vi "Import Structure from DB.vi"(8 "error in (no error)":errorcluster, 10 "Structure ID":string, 11 "connection reference":T2) -> (0 "error out":errorcluster, 2 "Loaded Structure":T1={"Structure Name"="Batch6_3+111 Quasi-Bulk", "Lattice vector a"=[9.1641, 0.0, 0.0], "Lattice vector b"=[0.0, 7.93635, 0.0], "Lattice vector c"=[0.0, 0.0, 53.7091], "Atoms Array"=[{"Atom Name"="", "Positions (Direct)"=[[0.036896, 0.129554, 0.035254], [0.536896, 0.129554, 0.035254], [0.286896, 0.629554, 0.035254], [0.786896, 0.629554, 0.035254], [0.285415, 0.295133, 0.107673], [0.785415, 0.295133, 0.107673], [0.035415, 0.795133, 0.107673], [0.535415, 0.795133, 0.107673], [0.033615, 0.463308, 0.180101], [0.533615, 0.463308, 0.180101], [0.283615, 0.963308, 0.180101], [0.783615, 0.963308, 0.180101], [0.030844, 0.131453, 0.252535], [0.530844, 0.131453, 0.252535], [0.280844, 0.631453, 0.252535], [0.780844, 0.631453, 0.252535], [0.278379, 0.302058, 0.324923], [0.778379, 0.302058, 0.324923], [0.028379, 0.802058, 0.324923], [0.528379, 0.802058, 0.324923], [0.031198, 0.471844, 0.397363], [0.531198, 0.471844, 0.397363], [0.281198, 0.971844, 0.397363], [0.781198, 0.971844, 0.397363], [0.03247, 0.140643, 0.469814], [0.53247, 0.140643, 0.469814], [0.28247, 0.640643, 0.469814], [0.78247, 0.640643, 0.469814], [0.284308, 0.303948, 0.542263], [0.784308, 0.303948, 0.542263], [0.034308, 0.803948, 0.542263], [0.534308, 0.803948, 0.542263], [0.035944, 0.468219, 0.614701], [0.535944, 0.468219, 0.614701], [0.285944, 0.968219, 0.614701], [0.785944, 0.968219, 0.614701], [0.037813, 0.131858, 0.687216], [0.537813, 0.131858, 0.687216], [0.787813, 0.631858, 0.687216], [0.287813, 0.631858, 0.687216], [0.038238, 0.463759, 0.759817], [0.538238, 0.463759, 0.759817], [0.288238, 0.963758, 0.759817], [0.788238, 0.963758, 0.759817], [0.038639, 0.130134, 0.831025], [0.538639, 0.130134, 0.831025], [0.288639, 0.630134, 0.831025], [0.788639, 0.630134, 0.831025], [0.285712, 0.295024, 0.89873], [0.785712, 0.295024, 0.89873], [0.035712, 0.795024, 0.89873], [0.535712, 0.795024, 0.89873], [0.032596, 0.464879, 0.966384], [0.532596, 0.464879, 0.966384], [0.282596, 0.964879, 0.966384], [0.782596, 0.964879, 0.966384]], "Positions (Cartesian)"=[[0.33811863359999994, 1.0281858879, 1.8934606114], [4.9201686336, 1.0281858879, 1.8934606114], [2.6291436335999996, 4.9963608879, 1.8934606114], [7.2111936336, 4.9963608879, 1.8934606114], [2.6155716014999997, 2.34227878455, 5.7830199243000004], [7.197621601499999, 2.34227878455, 5.7830199243000004], [0.3245466015, 6.31045378455, 5.7830199243000004], [4.9065966014999995, 6.31045378455, 5.7830199243000004], [0.30805122149999997, 3.6769744458, 9.673062619100001], [4.890101221499999, 3.6769744458, 9.673062619100001], [2.5990762215, 7.6451494458, 9.673062619100001], [7.1811262215, 7.6451494458, 9.673062619100001], [0.2826575004, 1.04325701655, 13.5634275685], [4.8647075004, 1.04325701655, 13.5634275685], [2.5736825004, 5.011432016550001, 13.5634275685], [7.155732500399999, 5.011432016550001, 13.5634275685], [2.5510929938999998, 2.3972380083, 17.4513218993], [7.1331429939, 2.3972380083, 17.4513218993], [0.2600679939, 6.3654130083, 17.4513218993], [4.8421179939000005, 6.3654130083, 17.4513218993], [0.28590159179999997, 3.7447191294, 21.3420091033], [4.867951591799999, 3.7447191294, 21.3420091033], [2.5769265918, 7.7128941294, 21.3420091033], [7.158976591799999, 7.7128941294, 21.3420091033], [0.29755832699999996, 1.11619207305, 25.2332871074], [4.879608327, 1.11619207305, 25.2332871074], [2.588583327, 5.08436707305, 25.2332871074], [7.170633327, 5.08436707305, 25.2332871074], [2.6054269428, 2.4122377098, 29.124457693300002], [7.1874769428, 2.4122377098, 29.124457693300002], [0.31440194279999994, 6.3804127098, 29.124457693300002], [4.8964519428, 6.3804127098, 29.124457693300002], [0.32939441039999995, 3.71594986065, 33.0150374791], [4.9114444104, 3.71594986065, 33.0150374791], [2.6204194104, 7.684124860650001, 33.0150374791], [7.202469410399999, 7.684124860650001, 33.0150374791], [0.3465221133, 1.0464712383, 36.909752865600005], [4.9285721133, 1.0464712383, 36.909752865600005], [7.2195971133, 5.0146462383, 36.909752865600005], [2.6375471132999997, 5.0146462383, 36.909752865600005], [0.3504168558, 3.6805537396499997, 40.809087234699994], [4.9324668557999995, 3.6805537396499997, 40.809087234699994], [2.6414418557999997, 7.6487208033, 40.809087234699994], [7.2234918558, 7.6487208033, 40.809087234699994], [0.35409165989999997, 1.0327889709, 44.6336048275], [4.9361416599, 1.0327889709, 44.6336048275], [2.6451166599, 5.0009639709, 44.6336048275], [7.227166659899999, 5.0009639709, 44.6336048275], [2.6182933392, 2.3414137224, 48.269979443000004], [7.200343339199999, 2.3414137224, 48.269979443000004], [0.3272683392, 6.3095887224, 48.269979443000004], [4.9093183391999995, 6.3095887224, 48.269979443000004], [0.29871300359999997, 3.6894424516499997, 51.9036148944], [4.880763003599999, 3.6894424516499997, 51.9036148944], [2.5897380036, 7.65761745165, 51.9036148944], [7.171788003599999, 7.65761745165, 51.9036148944]]}, {"Atom Name"="", "Positions (Direct)"=[[0.286795, 0.296109, 0.054458], [0.786795, 0.296109, 0.054458], [0.036795, 0.796109, 0.054458], [0.536795, 0.796109, 0.054458], [0.035258, 0.462031, 0.126878], [0.535258, 0.462031, 0.126878], [0.285258, 0.962031, 0.126878], [0.785258, 0.962031, 0.126878], [0.033445, 0.130094, 0.199309], [0.533445, 0.130094, 0.199309], [0.283445, 0.630094, 0.199309], [0.783445, 0.630094, 0.199309], [0.280766, 0.298203, 0.27171], [0.780766, 0.298203, 0.27171], [0.030766, 0.798203, 0.27171], [0.530766, 0.798203, 0.27171], [0.028505, 0.468822, 0.344121], [0.528505, 0.468822, 0.344121], [0.278505, 0.968822, 0.344121], [0.778505, 0.968822, 0.344121], [0.03126, 0.138635, 0.416572], [0.53126, 0.138635, 0.416572], [0.28126, 0.638635, 0.416572], [0.78126, 0.638635, 0.416572], [0.282556, 0.307128, 0.489026], [0.782556, 0.307128, 0.489026], [0.032556, 0.807128, 0.489026], [0.532556, 0.807128, 0.489026], [0.034374, 0.470438, 0.56147], [0.534374, 0.470438, 0.56147], [0.284374, 0.970438, 0.56147], [0.784374, 0.970438, 0.56147], [0.035964, 0.134698, 0.633895], [0.535964, 0.134698, 0.633895], [0.285964, 0.634698, 0.633895], [0.785964, 0.634698, 0.633895], [0.037794, 0.465111, 0.706493], [0.537794, 0.465111, 0.706493], [0.787794, 0.965111, 0.706493], [0.287794, 0.965111, 0.706493], [0.038181, 0.130274, 0.779081], [0.538181, 0.130274, 0.779081], [0.288181, 0.630273, 0.779081], [0.788181, 0.630273, 0.779081], [0.288548, 0.296604, 0.847022], [0.788548, 0.296604, 0.847022], [0.038548, 0.796604, 0.847022], [0.538548, 0.796604, 0.847022], [0.035661, 0.461866, 0.914714], [0.535661, 0.461866, 0.914714], [0.285661, 0.961866, 0.914714], [0.785661, 0.961866, 0.914714], [0.032517, 0.131341, 0.982331], [0.532517, 0.131341, 0.982331], [0.282517, 0.631341, 0.982331], [0.782517, 0.631341, 0.982331]], "Positions (Cartesian)"=[[2.6282180595, 2.35002466215, 2.9248901678], [7.2102680595, 2.35002466215, 2.9248901678], [0.3371930595, 6.31819966215, 2.9248901678], [4.9192430595, 6.31819966215, 2.9248901678], [0.32310783779999996, 3.66683972685, 6.814503189799999], [4.9051578378, 3.66683972685, 6.814503189799999], [2.6141328378, 7.63501472685, 6.814503189799999], [7.1961828377999995, 7.63501472685, 6.814503189799999], [0.3064933245, 1.0324715168999998, 10.704707011899998], [4.8885433245, 1.0324715168999998, 10.704707011899998], [2.5975183244999998, 5.000646516900001, 10.704707011899998], [7.179568324499999, 5.000646516900001, 10.704707011899998], [2.5729677006, 2.36664337905, 14.593299561], [7.155017700599999, 2.36664337905, 14.593299561], [0.2819427006, 6.33481837905, 14.593299561], [4.863992700599999, 6.33481837905, 14.593299561], [0.2612226705, 3.7207354797, 18.4824292011], [4.843272670499999, 3.7207354797, 18.4824292011], [2.5522476705, 7.6889104797, 18.4824292011], [7.1342976705, 7.6889104797, 18.4824292011], [0.286469766, 1.1002558822500002, 22.3737072052], [4.8685197659999995, 1.1002558822500002, 22.3737072052], [2.577494766, 5.0684308822499995, 22.3737072052], [7.159544765999999, 5.0684308822499995, 22.3737072052], [2.5893714396, 2.4374753028000002, 26.2651463366], [7.1714214396, 2.4374753028000002, 26.2651463366], [0.2983464396, 6.4056503028, 26.2651463366], [4.8803964396, 6.4056503028, 26.2651463366], [0.3150067734, 3.7335606213, 30.156048377], [4.8970567734, 3.7335606213, 30.156048377], [2.6060317734, 7.7017356213, 30.156048377], [7.1880817733999995, 7.7017356213, 30.156048377], [0.3295776924, 1.0690104723, 34.045929944499996], [4.9116276924, 1.0690104723, 34.045929944499996], [2.6206026924, 5.0371854723, 34.045929944499996], [7.202652692399999, 5.0371854723, 34.045929944499996], [0.3463479954, 3.69128368485, 37.9451031863], [4.928397995399999, 3.69128368485, 37.9451031863], [7.2194229953999995, 7.659458684850001, 37.9451031863], [2.6373729954, 7.659458684850001, 37.9451031863], [0.34989450209999995, 1.0339000599000001, 41.843739337100004], [4.9319445020999995, 1.0339000599000001, 41.843739337100004], [2.6409195021, 5.00206712355, 41.843739337100004], [7.2229695021, 5.00206712355, 41.843739337100004], [2.6442827268, 2.3539531553999997, 45.4927893002], [7.2263327268, 2.3539531553999997, 45.4927893002], [0.35325772679999995, 6.3221281554, 45.4927893002], [4.9353077268, 6.3221281554, 45.4927893002], [0.3268009701, 3.6655302291, 49.1284656974], [4.9088509701000005, 3.6655302291, 49.1284656974], [2.6178259700999997, 7.6337052291, 49.1284656974], [7.1998759701, 7.6337052291, 49.1284656974], [0.29798903969999996, 1.04236814535, 52.760113912099996], [4.8800390397, 1.04236814535, 52.760113912099996], [2.5890140397, 5.010543145350001, 52.760113912099996], [7.1710640397, 5.010543145350001, 52.760113912099996]]}], "# of atoms"=112}, 3 "connection reference out":T2)   [LabVIEW 2010]
uses:
  <vilib>/addons/database/Connection.llb/Conn ObjectReference.ctl
  <vilib>/addons/database/_DB Variant To Data/Database Variant To Data.xnode
  <vilib>/addons/database/NI_Database_API.lvlib
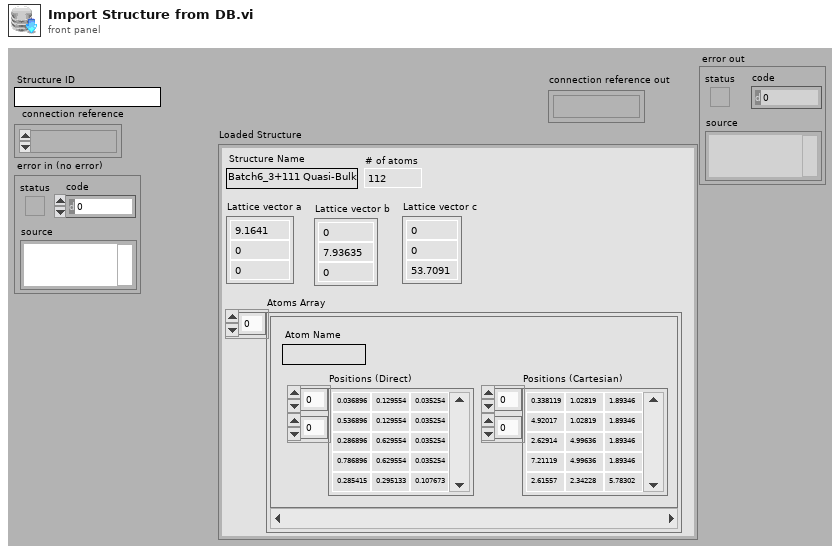
[diagram p1: front panel]
types:
  T1 = cluster{"Structure Name":string, "Lattice vector a":dbl[], "Lattice vector b":dbl[], "Lattice vector c":dbl[], "Atoms Array":cluster{"Atom Name":string, "Positions (Direct)":dbl[][], "Positions (Cartesian)":dbl[][]}[], "# of atoms":i32}
  T2 = typedef "NI_Database_API.lvlib/Conn ObjectReference.ctl" = refnum<k1>
  T3 = cluster{"Atom Name":string, "Positions (Direct)":dbl[][], "Positions (Cartesian)":dbl[][]}
  T4 = cluster{"Atom Name":string, "Positions (Direct)":dbl[][], "Positions (Cartesian)":dbl[][]}[]
  T5 = cluster{"data":string, dbl[], dbl[], dbl[], cluster{"Atom Name":string, "Positions (Direct)":dbl[][], "Positions (Cartesian)":dbl[][]}[], "data":dbl}
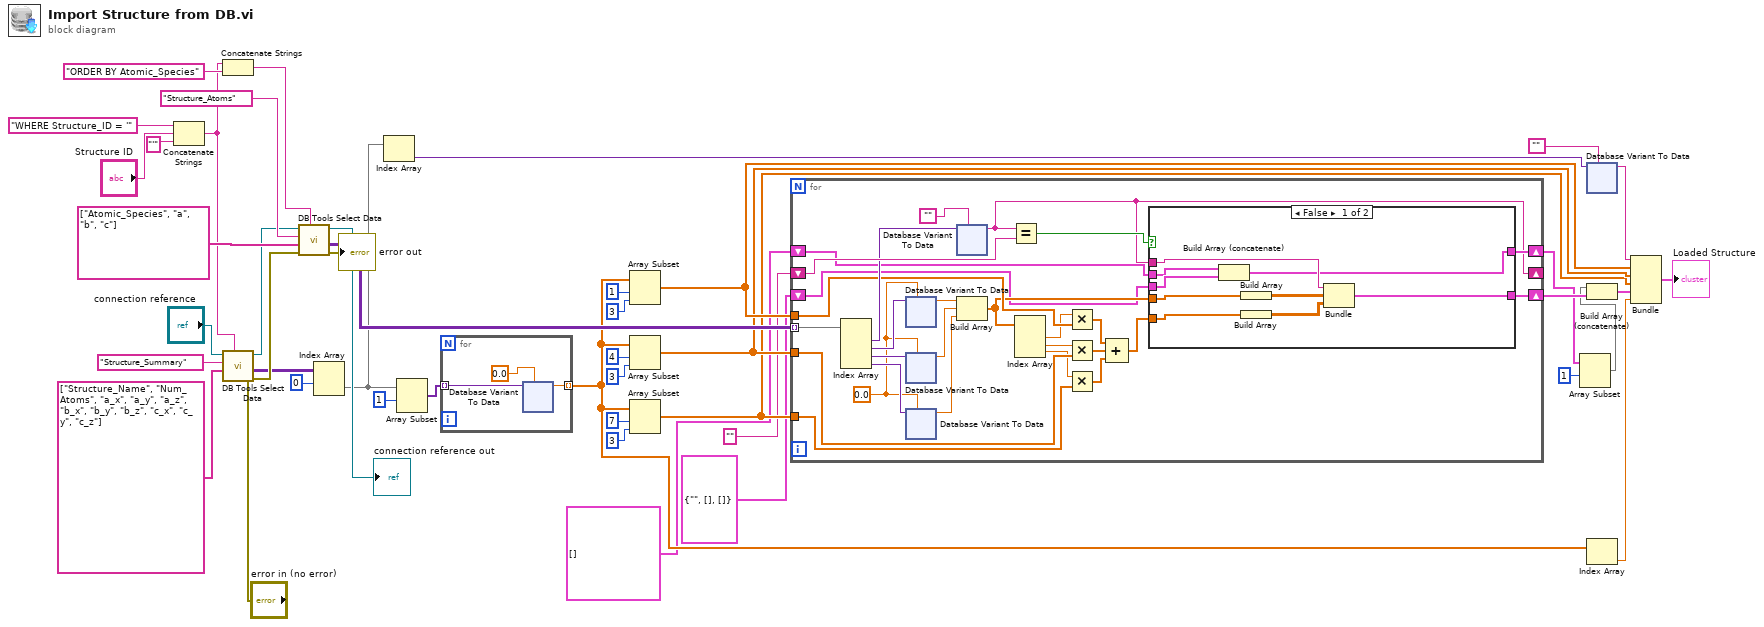
[diagram p0: block diagram]
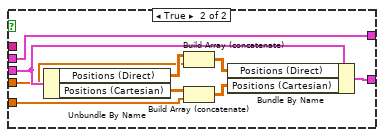
[diagram p2: hidden frame]
diagram:
  n1 = Concatenate Strings("WHERE Structure_ID = '", "Structure ID", "'" ("string")) -> (w19:string)
  n2 = Concatenate Strings(w19, "ORDER BY Atomic_Species" ("string")) -> (w18:string)
  n3 = call <vilib>:"DB Tools Select Data.vi"("condition"=w19, "error in (no error)"="error in (no error)", "columns"=string[] ["Structure_Name", "Num_Atoms", "a_x", "a_y", "a_z", "b_x", "b_y", "b_z", "c_x", "c_y", "c_z"], "table"="Structure_Summary", "connection reference"="connection reference") -> ("error out"=w34:errorcluster, "data"=w33:variant[][], "connection reference out"=w40:T2)  [unwired: 1 in]
  n4 = call <vilib>:"DB Tools Select Data.vi"("condition"=w18, "error in (no error)"=w34, "columns"=string[] ["Atomic_Species", "a", "b", "c"], "table"="Structure_Atoms", "connection reference"=w40) -> ("error out"=→"error out":errorcluster, "data"=w43:variant[][], "connection reference out"=→"connection reference out":T2)  [unwired: 1 in]
  n5 = Index Array(array=w33, index (row)=0) -> (element=w8:variant[])  [unwired: 1 in]
  n6 = Index Array(array=w8) -> (element=w31:variant)  [unwired: 1 in]
  n7 = Array Subset(array=w8, index=1) -> (w9:variant[])  [unwired: 1 in]
  n8 = for {
    tunnel: w9 -> [w48] mode=indexing
    tunnel: [w47] -> w23 mode=indexing
    n9 = xnode "Database Variant To Data"("database variant"=w48, "type"=0.0) -> ("data"=w47:dbl)  [unwired: 1 in, 1 out]
  }
  n10 = Array Subset(array=w23, index=1, length=3) -> (w16:dbl[])
  n11 = Array Subset(array=w23, index=4, length=3) -> (w15:dbl[])
  n12 = Array Subset(array=w23, index=7, length=3) -> (w14:dbl[])
  n13 = for {
    tunnel: w43 -> [w107] mode=indexing
    shift-right: [w81] -> _
    shift-left: "" ("data") -> [w108]
    tunnel: w16 -> [w97]
    tunnel: w15 -> [w96]
    tunnel: w14 -> [w95]
    shift-right: [w83] -> w5
    shift-left: T4 [] ("Atoms Array") -> [w82]
    shift-right: [w85] -> w13
    shift-left: T3 {"Atom Name"="", "Positions (Direct)"=[], "Positions (Cartesian)"=[]} ("Atomic Positions") -> [w84]
    w101 = 0.0
    n14 = Index Array(array=w107) -> (element #1=w106:variant, element #2=w104:variant, element #3=w103:variant, element #4=w102:variant)  [unwired: 4 in]
    n15 = xnode "Database Variant To Data"("database variant"=w104, "type"=w101) -> ("data"=w100:dbl)  [unwired: 1 in, 1 out]
    n16 = xnode "Database Variant To Data"("database variant"=w103, "type"=w101) -> ("data"=w99:dbl)  [unwired: 1 in, 1 out]
    n17 = xnode "Database Variant To Data"("database variant"=w102, "type"=w101) -> ("data"=w98:dbl)  [unwired: 1 in, 1 out]
    n18 = xnode "Database Variant To Data"("database variant"=w106, "type"="") -> ("data"=w81:string)  [unwired: 1 in, 1 out]
    n19 = Build Array(w100, w99, w98) -> (w86:dbl[])
    n20 = Equal?(x=w81, y=w108) -> (x = y?=w88:bool)
    n21 = Index Array(array=w86) -> (element #1=w89:dbl, element #2=w90:dbl, element #3=w91:dbl)  [unwired: 3 in]
    n22 = Multiply(x=w89, y=w97) -> (x*y=w92:dbl[])
    n23 = Multiply(x=w90, y=w96) -> (x*y=w93:dbl[])
    n24 = Multiply(x=w91, y=w95) -> (x*y=w94:dbl[])
    n25 = Compound Arithmetic op=ADD(w92, w93, w94) -> (w87:dbl[])
    n26 = case shown="False" w88 {
      tunnel: w87 -> [w115 w120]
      tunnel: w86 -> [w116 w123]
      tunnel: w81 -> [w117 _]
      tunnel: [w112 w118] -> w85
      tunnel: w84 -> [w111 w125]
      tunnel: [w110 w126] -> w83
      tunnel: w82 -> [w109 w126]
      frame False {
        n27 = Build Array (concatenate)(w109, w111) -> (w110:T4)
        n28 = Build Array(w116) -> (w114:dbl[][])
        n29 = Build Array(w115) -> (w113:dbl[][])
        n30 = Bundle("data"=w117, w114, w113) -> (w112:cluster{"data":string, dbl[][], dbl[][]})  [unwired: 1 in]
      }
      frame True {
        n31 = Unbundle By Name(w125) -> ("Positions (Direct)"=w124:dbl[][], "Positions (Cartesian)"=w121:dbl[][])
        n32 = Build Array (concatenate)(w124, w123) -> (w122:dbl[][])
        n33 = Build Array (concatenate)(w121, w120) -> (w119:dbl[][])
        n34 = Bundle By Name(cluster=w125, "Positions (Direct)"=w122, "Positions (Cartesian)"=w119) -> (w118:T3)
      }
    }
  }
  n35 = Array Subset(array=w5, index=1) -> (w3:T4)  [unwired: 1 in]
  n36 = xnode "Database Variant To Data"("database variant"=w31, "type"="") -> ("data"=w22:string)  [unwired: 1 in, 1 out]
  n37 = Build Array (concatenate)(w3, w13) -> (w12:T4)
  n38 = Index Array(array=w23) -> (element=w21:dbl)  [unwired: 1 in]
  n39 = Bundle("data"=w22, w16, w15, w14, w12, "data"=w21) -> (→"Loaded Structure":T5)  [unwired: 1 in]
